vi "StopAndClearAllCache.vi"(5 "error in (no error)":errorcluster) -> (19 "error out":errorcluster)   [LabVIEW 2020, in "DP_WebView.lvclass"]
uses:
  DP_WebView.lvclass
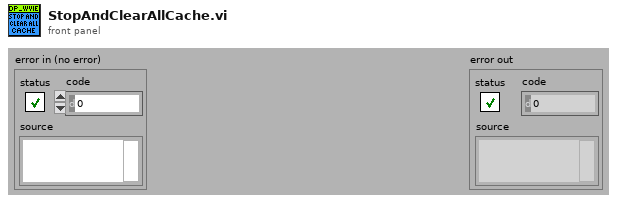
[diagram p1: front panel]
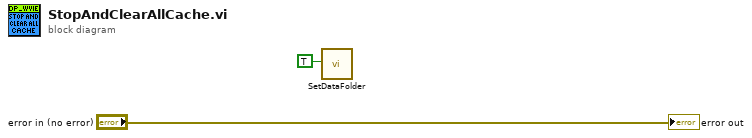
[diagram p0: block diagram]
diagram:
  n1 = call "SetDataFolder.vi"("JustKillAllSavedReferences(False)"=TRUE) -> ()  [unwired: 15 in, 4 out]
  "error out" <- "error in (no error)"
